vi "coerce exposure to available increment.vi"(6 "desired exposure":dbl, 9 "Increment":dbl, 10 "Min":dbl, 11 "Max":dbl) -> (3 "closest available exposure":dbl)   [LabVIEW 2020]
panel:
  out "floor(x/y)":dbl
  out "x-y*floor(x/y)":dbl
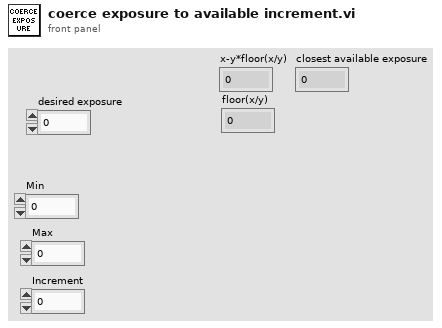
[diagram p1: front panel]
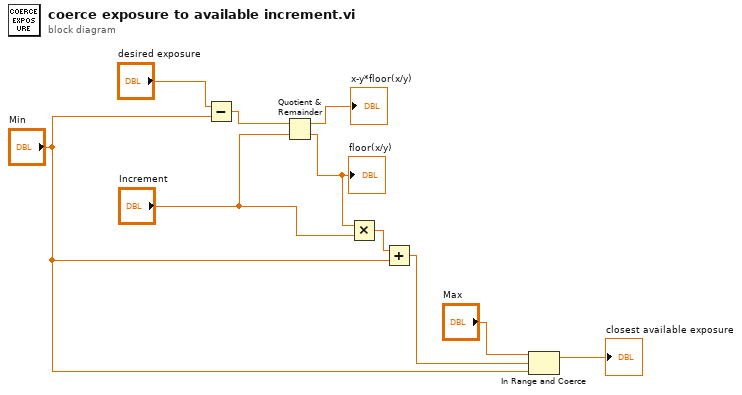
[diagram p0: block diagram]
diagram:
  n1 = Subtract(x="desired exposure", y="Min") -> (x-y=w9:dbl)
  n2 = Quotient & Remainder(x=w9, y="Increment") -> (x-y*floor(x/y)=→"x-y*floor(x/y)":dbl, floor(x/y)=w7:dbl)
  "floor(x/y)" <- w7
  n3 = Multiply(x=w7, y="Increment") -> (x*y=w5:dbl)
  n4 = Add(x=w5, y="Min") -> (x+y=w3:dbl)
  n5 = In Range and Coerce(upper limit="Max", x=w3, lower limit="Min") -> (coerced(x)=→"closest available exposure":dbl)  [unwired: 1 out]
